vi "Box Width SubVI.vi"(0 "Image":T4, 5 "Coord details":T5, 7 "Calibrated Image":T4, 11 "error in (no error)":errorcluster, 12 "M ROI":T7) -> (4 "Image Out":T4, 6 "Box Width":sgl, 10 "All Edges":T6, 15 "error out":errorcluster)   [LabVIEW 2019, in "Algorithm.lvclass"]
uses:
  FrameworkOverrides/Algorithm.lvclass
  <vilib>/vision/Measure.llb/Search Line.ctl
  <vilib>/vision/Measure.llb/Edge New.ctl
  <vilib>/vision/Measure.llb/Edge Options.ctl
  <vilib>/vision/Measure.llb/Edge Polarity.ctl
  <vilib>/vision/NI_Vision_Development_Module.lvlib
  <vilib>/vision/Image Controls.llb/IMAQ Image.ctl
panel:
  out "Overlay Cluster out":T3 {"Search Lines"."Edge Info"."Distance (Real-World)" format="%.2f"; "Search Lines"."Edge Info"."Location (Real-World)"."Y" format="%.2g"; "Search Lines"."Edge Info"."Location (Real-World)"."X" format="%.2f"; "Search Lines"."Edge Info"."Noise" format="%.2f"; "Search Lines"."Edge Info"."Location (Pixel)"."Y" format="%.2g"; "Search Lines"."Edge Info"."Location (Pixel)"."X" format="%.2f"; "Search Lines"."Edge Info"."Strength" format="%.2f"; "Search Lines"."Edge Info"."Distance (Pixel)" format="%.2f"}
  out "Angle (Pixel)":dbl
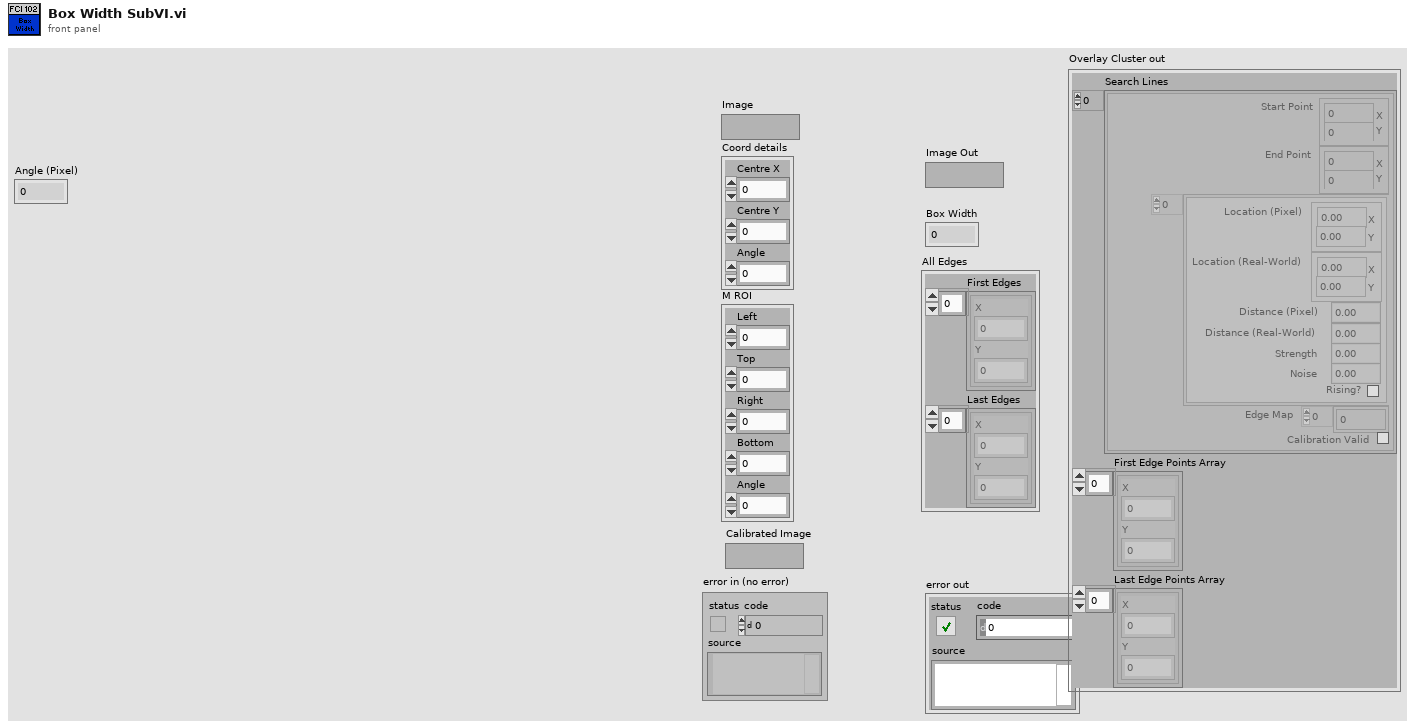
[diagram p1: front panel]
types:
  T1 = typedef "Search Line.ctl" = cluster{"Start Point":cluster{"X":sgl, "Y":sgl}, "End Point":cluster{"X":sgl, "Y":sgl}, "Edge Info":T2[], "Edge Map":dbl[], "Calibration Valid":bool}
  T2 = typedef "Edge New.ctl" = cluster{"Location (Pixel)":cluster{"X":sgl, "Y":sgl}, "Location (Real-World)":cluster{"X":sgl, "Y":sgl}, "Distance (Pixel)":dbl, "Distance (Real-World)":dbl, "Strength":dbl, "Noise":dbl, "Rising?":bool}
  T3 = cluster{"Search Lines":T1[], "First Edge Points Array":cluster{"X":sgl, "Y":sgl}[], "Last Edge Points Array":cluster{"X":sgl, "Y":sgl}[]}
  T4 = typedef "IMAQ Image.ctl" = refnum<image>
  T5 = cluster{"Centre X":dbl, "Centre Y":dbl, "Angle":dbl}
  T6 = cluster{"First Edges":cluster{"X":sgl, "Y":sgl}[], "Last Edges":cluster{"X":sgl, "Y":sgl}[]}
  T7 = cluster{"Left":dbl, "Top":dbl, "Right":dbl, "Bottom":dbl, "Angle":dbl}
  T8 = enum16{"Get First Edge", "Get First + Last Edge", "Get All Edges", "Get Best Edge"}
  T9 = typedef "Edge Options.ctl" = cluster{"Edge Polarity":T10, "Kernel Size":u32, "Width":u32, "Minimum Edge Strength":sgl, "Interpolation Type":enum32{"Zero Order", "Bilinear", "Quadratic", "Cubic", "Bilinear Fixed"}, "Data Processing Method":enum32{"Average", "Median"}}
  T10 = typedef "Edge Polarity.ctl" = u32
  T11 = typedef "ROI Descriptor" = cluster{"Global Rectangle":i32[], "Contours":cluster{"ID":enum32{"External", "Internal"}, "Type":u32, "Coordinates":i32[]}[]}
  T12 = cluster{"First Edge Point":cluster{"X":sgl, "Y":sgl}, "Search Line First Edge":cluster{"X":sgl, "Y":sgl}}
  T13 = cluster{"Last Edge Point":cluster{"X":sgl, "Y":sgl}, "Search Line Last Edge":cluster{"X":sgl, "Y":sgl}}
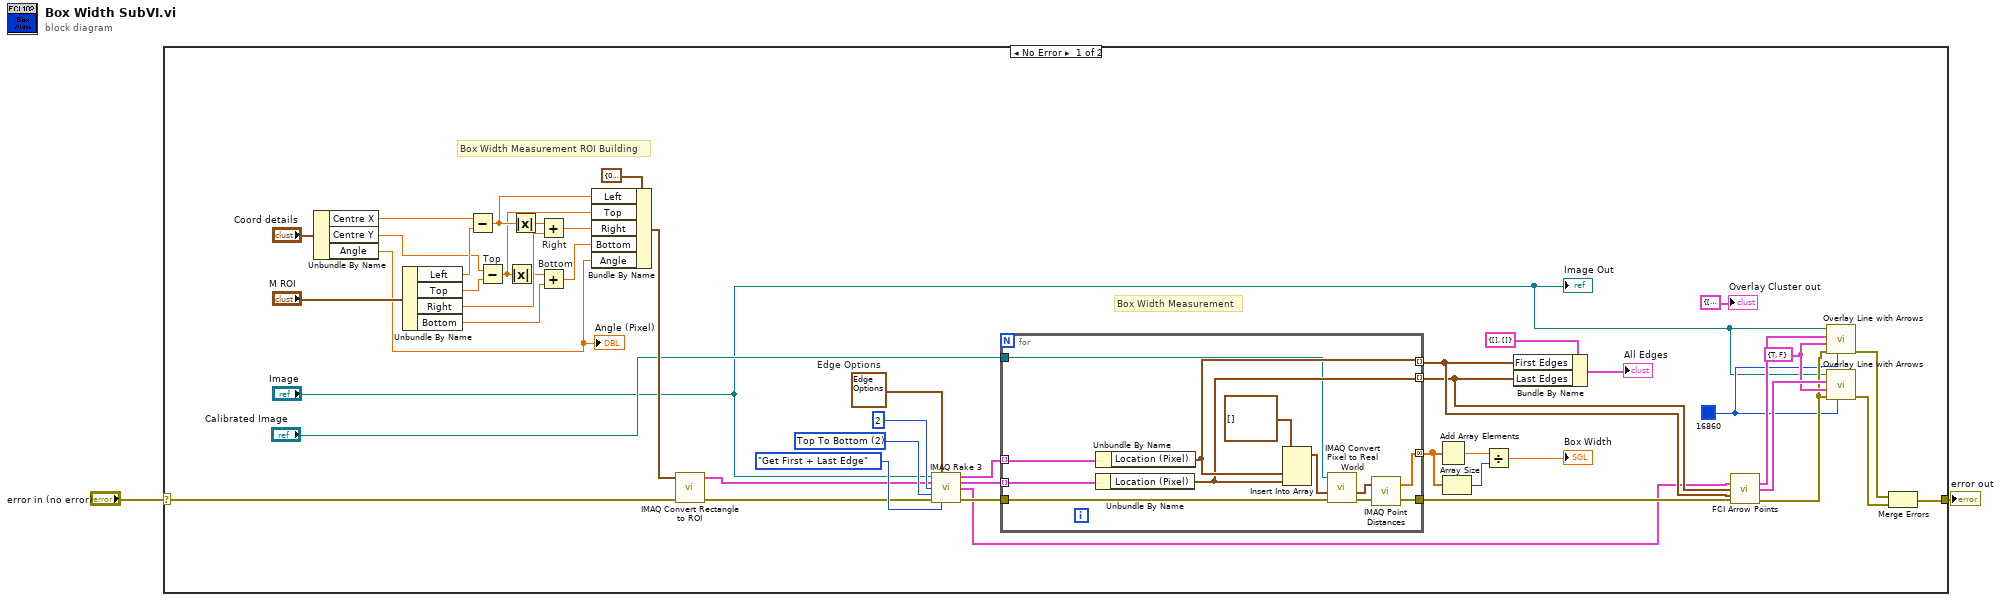
[diagram p0: block diagram]
diagram:
  n1 = case shown="No Error" "error in (no error)" {
    selector: "error in (no error)" -> [w19 w63]
    tunnel: [w5 w63] -> w1
    frame No Error {
      w12 = u32 16860 ("Color")
      w14 = cluster{"Start point":bool, "End point":bool} {"Start point"=TRUE, "End point"=FALSE} ("Arrows")
      w38 = T9 {"Edge Polarity"=0, "Kernel Size"=5, "Width"=5, "Minimum Edge Strength"=50.0, "Interpolation Type"=enum."Zero Order", "Data Processing Method"=enum."Average"}  # Edge Options
      w40 = u16 2 items=["Left To Right", "Right To Left", "Top To Bottom", "Bottom To Top"] ("Scan Direction")
      # "Box Width Measurement"
      # "Box Width Measurement ROI Building"
      n2 = Unbundle By Name("Coord details") -> ("Centre X"=w22:dbl, "Centre Y"=w21:dbl, "Angle"=w20:dbl)
      "Angle (Pixel)" <- w20
      n3 = Unbundle By Name("M ROI") -> ("Left"=w45:dbl, "Top"=w44:dbl, "Right"=w43:dbl, "Bottom"=w42:dbl)
      n4 = Subtract(x=w22, y=w45) -> (x-y=w48:dbl)
      n5 = Subtract "Top"(x=w21, y=w44) -> (x-y=w31:dbl)
      n6 = Absolute Value(x=w31) -> (abs(x)=w32:dbl)
      n7 = Absolute Value(x=w48) -> (abs(x)=w50:dbl)
      n8 = Add "Right"(x=w50, y=w43) -> (x+y=w47:dbl)
      n9 = Add "Bottom"(x=w32, y=w42) -> (x+y=w46:dbl)
      n10 = Bundle By Name(cluster=T7 {"Left"=0.0, "Top"=0.0, "Right"=0.0, "Bottom"=0.0, "Angle"=0.0} ("input cluster"), "Left"=w48, "Top"=w31, "Right"=w47, "Bottom"=w46, "Angle"=w20) -> (w33:T7)
      n11 = call "IMAQ Convert Rectangle to ROI"("error in (no error)"=w19, "Rectangle"=w33) -> ("error out"=w29:errorcluster, "ROI Descriptor"=w30:T11)  [unwired: 7 in]
      n12 = call "IMAQ Rake 3"("Image"="Image", "Edge Options"=w38, "ROI Descriptor"=w30, "Step Size"=u32 2, "Scan Direction"=w40, "error in (no error)"=w29, "Process"=T8."Get First + Last Edge") -> ("First Edges"=w26:T2[], "Last Edges"=w8:T2[], "Search Lines"=w7:T1[], "error out"=w28:errorcluster)  [unwired: 5 in]
      n13 = for {
        tunnel: w26 -> [w62] mode=indexing
        tunnel: w8 -> [w61] mode=indexing
        tunnel: [w59] -> w37 mode=concatenating
        tunnel: w28 -> [w52]
        tunnel: [w58] -> w11
        tunnel: [w56] -> w10 mode=indexing
        tunnel: [w55] -> w9 mode=indexing
        tunnel: "Calibrated Image" -> [w53]
        n14 = Unbundle By Name(w61) -> ("Location (Pixel)"=w55:cluster{"X":sgl, "Y":sgl})
        n15 = Unbundle By Name(w62) -> ("Location (Pixel)"=w56:cluster{"X":sgl, "Y":sgl})
        n16 = Insert Into Array(array=cluster{"X":sgl, "Y":sgl}[] [], new element #1=w56, new element #2=w55) -> (w57:cluster{"X":sgl, "Y":sgl}[])  [unwired: 1 in]
        n17 = call "IMAQ Convert Pixel to Real World"("error in (no error)"=w52, "Array of Pixel Coordinates"=w57, "Calibrated Image"=w53) -> ("error out"=w51:errorcluster, "Array of Real World Coordinates"=w54:cluster{"X":sgl, "Y":sgl}[])  [unwired: 3 in, 4 out]
        n18 = call "IMAQ Point Distances"("Points"=w54, "error in (no error)"=w51) -> ("Distances"=w59:sgl[], "error out"=w58:errorcluster)  [unwired: 3 in]
      }
      n19 = Add Array Elements(numeric array=w37) -> (sum=w36:sgl)
      n20 = Array Size(array=w37) -> (size(s)=w35:i32)
      n21 = Divide(x=w36, y=w35) -> (x/y=→"Box Width":sgl)
      n22 = Bundle By Name(cluster=T6 {"First Edges"=[], "Last Edges"=[]} ("All Edges"), "First Edges"=w10, "Last Edges"=w9) -> (→"All Edges":T6)
      n23 = call "FCI Arrow Points.vi"("Search Lines"=w7, "Edge Last Points"=w9, "Edge First Points"=w10, "error constant"=w11) -> ("First Arrow Line Coord"=w16:T12, "Second Arrow Line Coord"=w15:T13, "error IO"=w13:errorcluster)  [unwired: 7 in, 2 out]
      n24 = call <vilib>:"Overlay Line with Arrows.vi"("Color"=w12, "error in (no error)"=w13, "Arrows"=w14, "Line Coordinates"=w16, "Image In"="Image") -> ("error out"=w4:errorcluster)  [unwired: 5 in, 1 out]
      n25 = call <vilib>:"Overlay Line with Arrows.vi"("Color"=w12, "error in (no error)"=w13, "Arrows"=w14, "Line Coordinates"=w15, "Image In"="Image") -> ("error out"=w3:errorcluster)  [unwired: 5 in, 1 out]
      n26 = Merge Errors(w4, w3) -> (w5:errorcluster)
      "Image Out" <- "Image"
      "Overlay Cluster out" <- T3 {"Search Lines"=[], "First Edge Points Array"=[], "Last Edge Points Array"=[]} ("Overlay Cluster out")
    }
    frame Error {
    }
  }
  "error out" <- w1
